vi "Tosca-Setup Imaging.vi"(0 "Imaging In":T1, 1 "Parent VI":refnum<vi>) -> (4 "Imaging Out":T1, 8 "Canceled?":bool)   [LabVIEW 2020]
uses:
  Typedefs/Tosca-Imaging.ctl
  Imaging VIs/Tosca-Imaging Mode.ctl
  Imaging VIs/Tosca-2P Config.ctl
  Sub VIs/Tosca-Globals.vi
panel:
  in  "Mode":enum16{"Off", "Widefield", "Two-photon"}(ring)
  in  "Tab Control":enum32{"Off", "Widefield", "Two-photon"}(tab)
  in  "Frame trigger":enum16{"Digital output", "Analog output"}(ring)
  in  "Destination":u16(ring) items=["Signal 1", "Frame Out", "Signal 2"]
  in  "Frame rate":dbl format="%#_g Hz"
  in  "TrigSrc":u16(ring) caption="Trigger source" items=["Default", "/PXI1Slot2/PFI0", "/PXI1Slot3/PFI0", "/PXI1Slot3/PFI1", "/PXI1Slot3/PFI2", "/PXI1Slot3/PFI3", "/PXI1Slot3/PFI4", "/PXI1Slot3/PFI5", "/PXI1Slot3/PFI6", "/PXI1Slot3/PFI7", "/PXI1Slot3/PFI8", "/PXI1Slot3/PFI9", "/PXI1Slot3/PFI10", "/PXI1Slot3/PFI11", "/PXI1Slot3/PFI12", "/PXI1Slot3/PFI13", "/PXI1Slot3/PFI14", "/PXI1Slot3/PFI15", "/PXI1Slot4/PFI0", "/PXI1Slot4/PFI1", "/PXI1Slot4/PFI2", "/PXI1Slot4/PFI3", "/PXI1Slot4/PFI4", "/PXI1Slot4/PFI5", "/PXI1Slot4/PFI6", "/PXI1Slot4/PFI7", "/PXI1Slot4/PFI8", "/PXI1Slot4/PFI9", "/PXI1Slot4/PFI10", "/PXI1Slot4/PFI11", "/PXI1Slot4/PFI12", "/PXI1Slot4/PFI13", "/PXI1Slot4/PFI14", "/PXI1Slot4/PFI15"]
  in  "Terminal":u16(ring) items=["Default", "PFI0", "PFI1", "PFI2", "PFI3", "PFI4", "PFI5", "PFI6", "PFI7", "PFI8", "PFI9", "PFI10", "PFI11", "PFI12", "PFI13", "PFI14", "PFI15"]
  in  "Device":u16(ring) caption="Frame tracker" items=["PXI1Slot3", "PXI1Slot4"]
  out "exit signal":bool
  in  "Cancel":bool
  in  "OK":bool
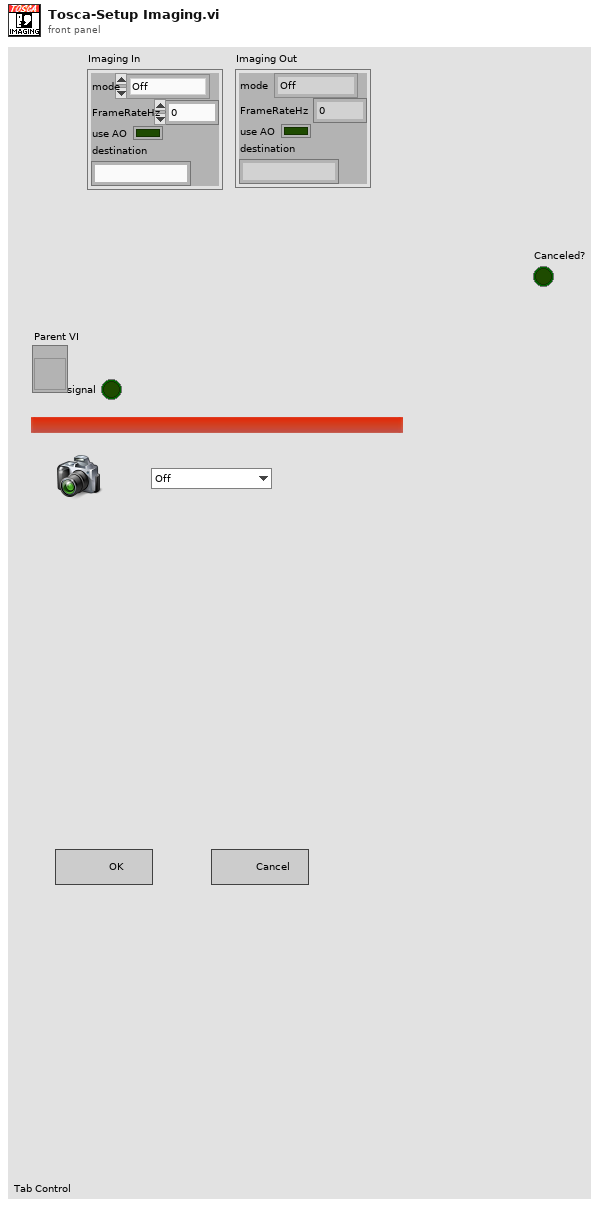
[diagram p1: front panel]
types:
  T1 = typedef "Tosca-Imaging.ctl" = cluster{"mode":T2, "FrameRateHz":dbl, "use AO":bool, "destination":string}
  T2 = typedef "Tosca-Imaging Mode.ctl" = enum16{"Off", "Widefield", "Two-photon"}
  T3 = typedef "Tosca-2P Config.ctl" = cluster{"Frame tracker":string, "Terminal":string, "Trigger source":string}
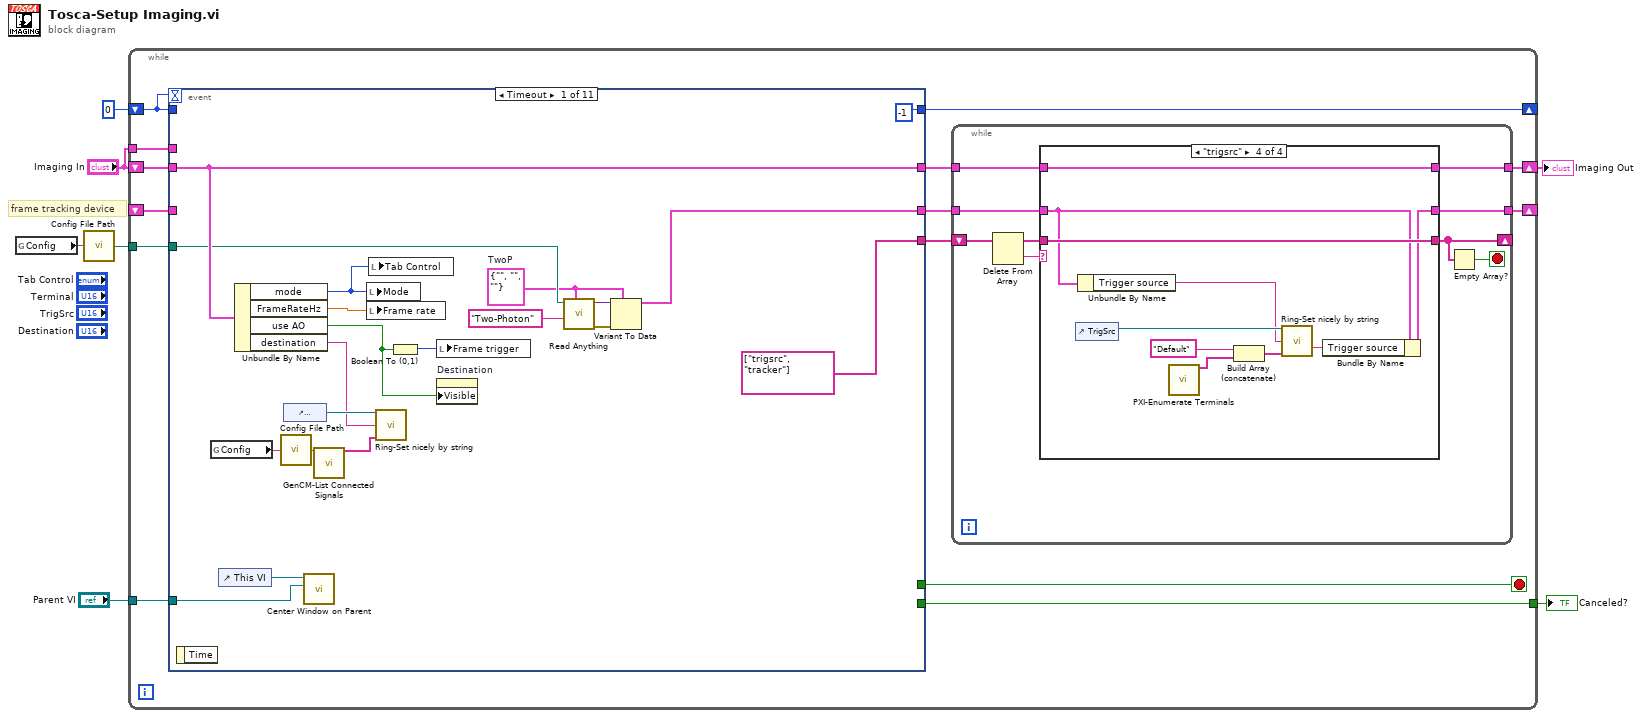
[diagram p0: block diagram]
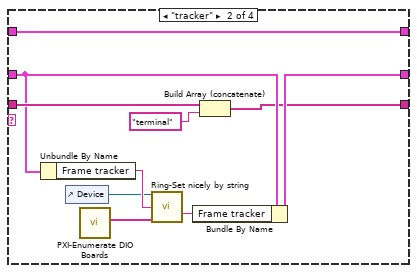
[diagram p3: hidden frame]
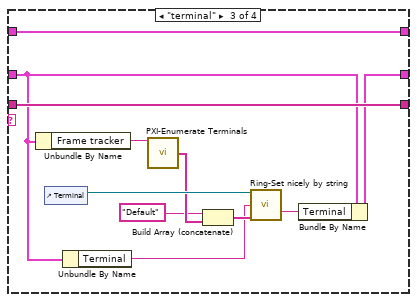
[diagram p4: hidden frame]
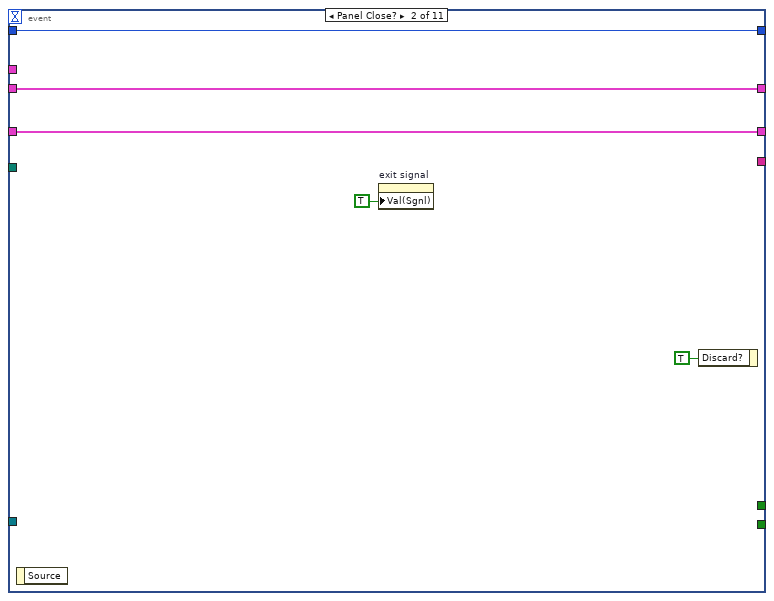
[diagram p5: hidden frame]
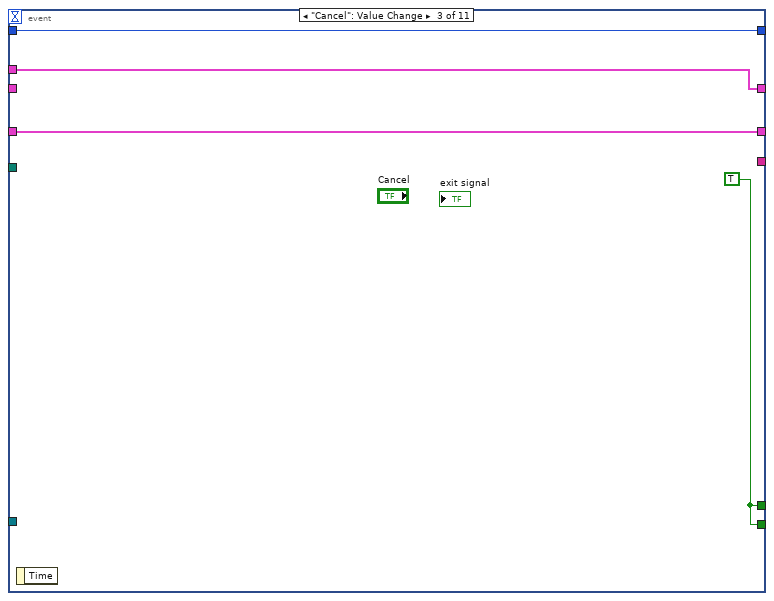
[diagram p6: hidden frame]
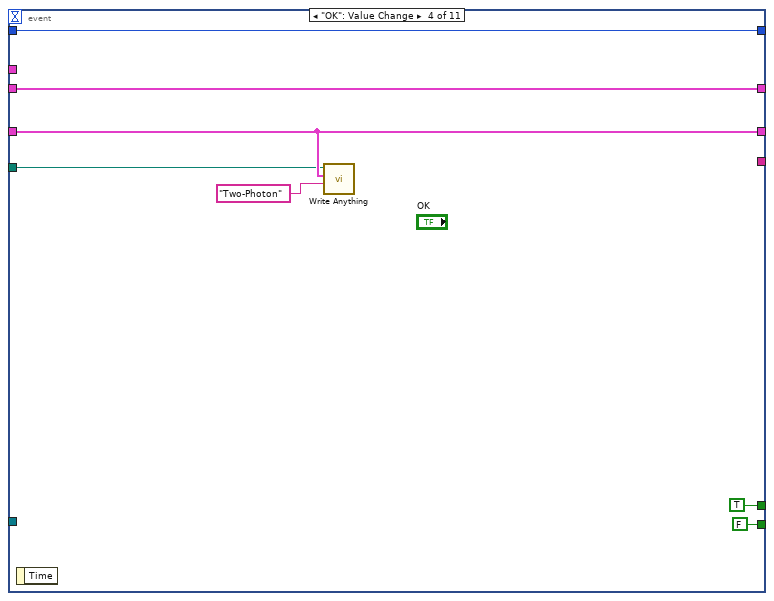
[diagram p7: hidden frame]
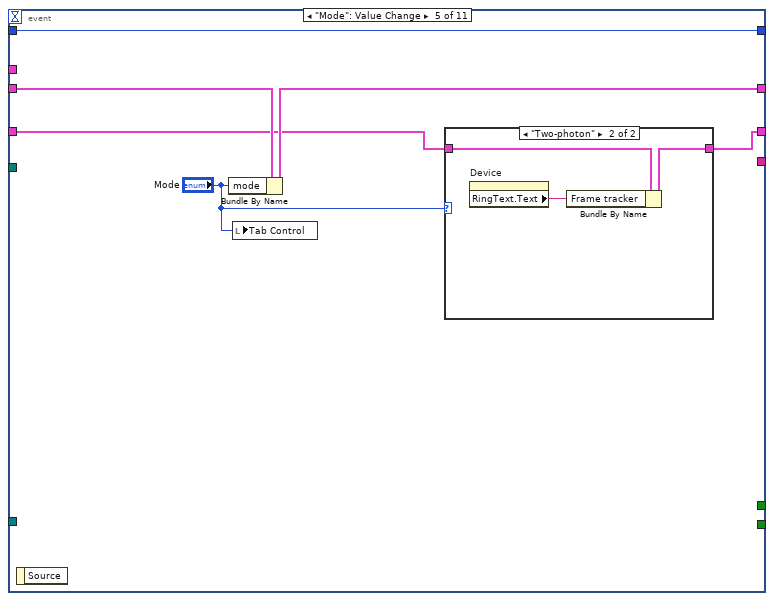
[diagram p8: hidden frame]
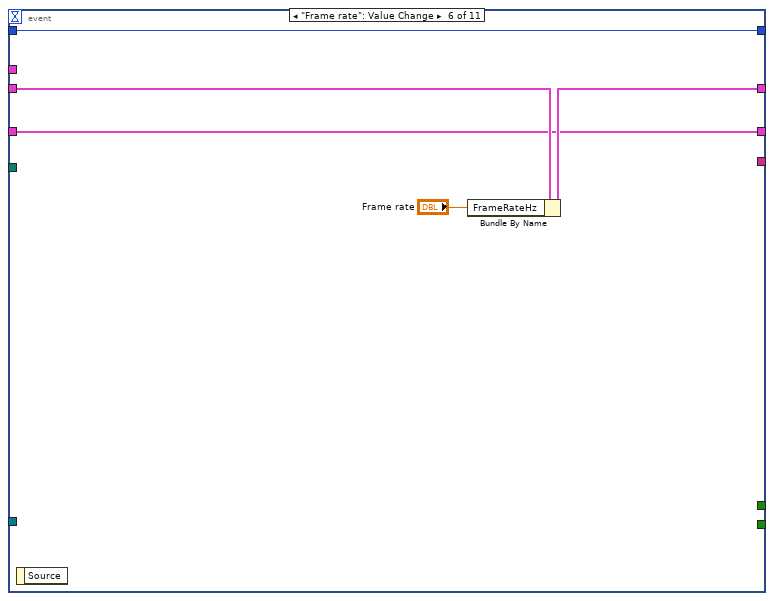
[diagram p10: hidden frame]
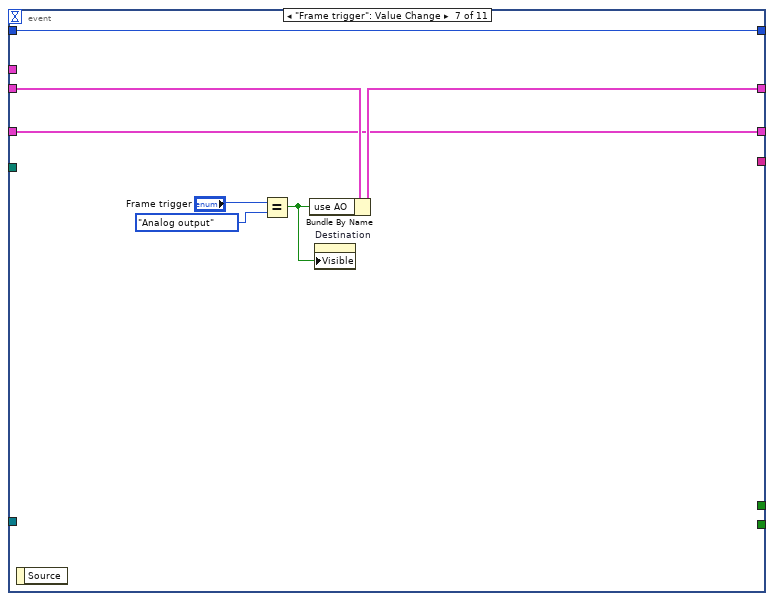
[diagram p11: hidden frame]
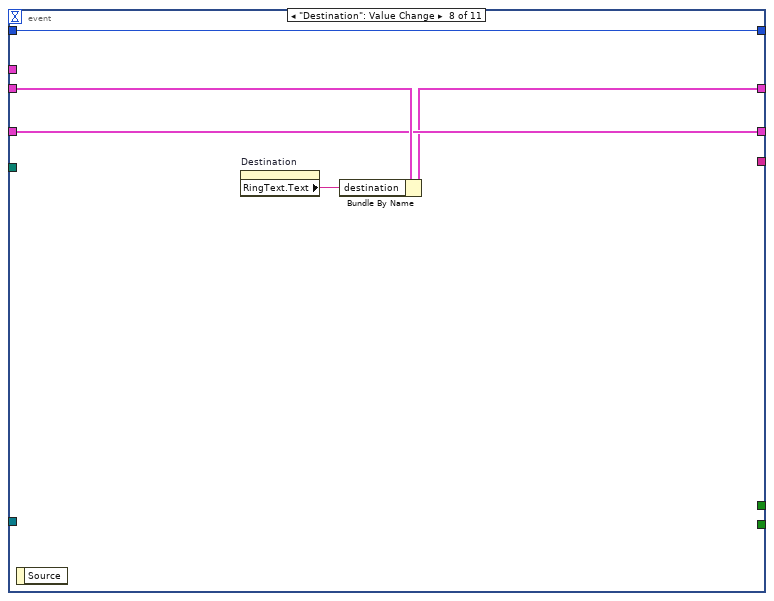
[diagram p12: hidden frame]
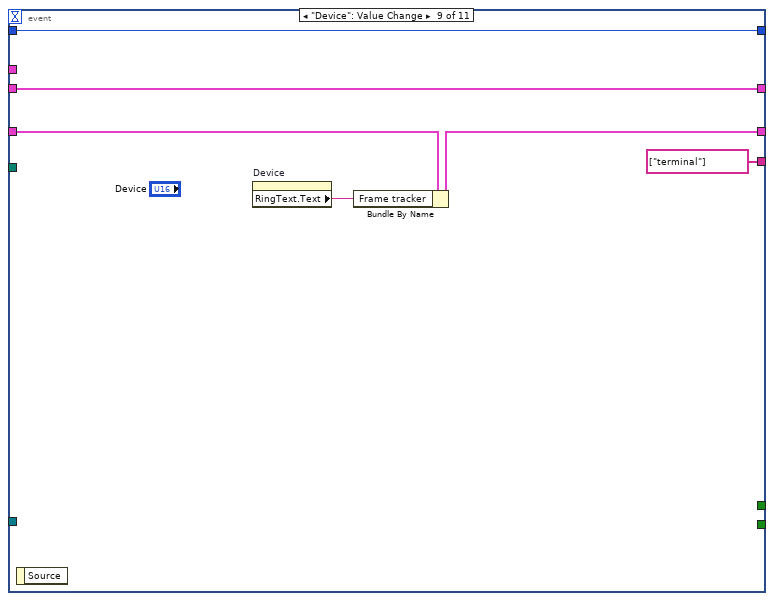
[diagram p13: hidden frame]
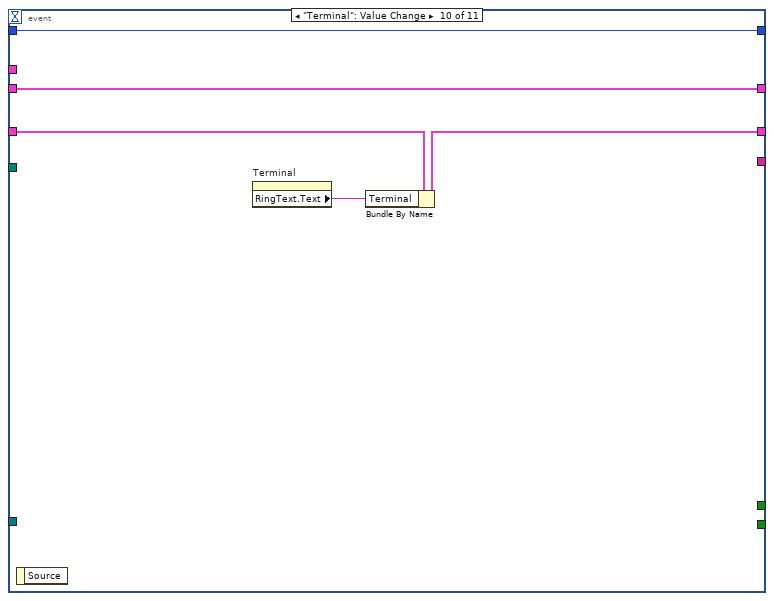
[diagram p14: hidden frame]
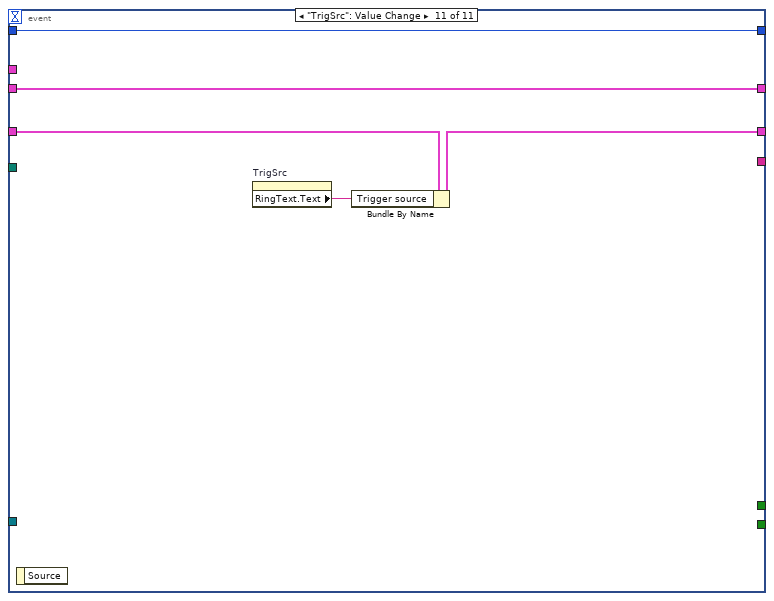
[diagram p15: hidden frame]
diagram:
  # "frame tracking device"
  n1 = global read "Tosca-Globals.vi" "Config"() -> (w1:string)
  n2 = call "Config File Path.vi"("AppName"=w1) -> ("Default config file name"=w4:path)
  n3 = while {
    shift-right: [w21] -> _
    shift-left: 0 -> [w17]
    tunnel: [w19] -> w5
    shift-right: [w12] -> w6
    shift-left: "Imaging In" -> [w18]
    tunnel: w4 -> [w8]
    shift-right: [w11] -> _
    shift-left: _ -> [w16]
    tunnel: "Imaging In" -> [w15]
    tunnel: "Parent VI" -> [w9]
    stop <- w20 stop-if-true
    n4 = event shown="[0] Timeout" {
      selector: _ -> [_ _ _ _ _ _ _ _ _ _ _]
      dyn-events: _ -> [_ _ _ _ _ _ _ _ _ _ _]
      timeout: w17 -> [_ _ _ _ _ _ _ _ _ _ _]
      tunnel: [-1 w89 w91 w97 w106 w115 w122 w127 w133 w138 w143] -> w21
      tunnel: w18 -> [w83 w88 _ w100 w105 w114 w121 w126 w132 w137 w142]
      tunnel: [w83 w88 w92 w100 w104 w113 w120 w124 w132 w137 w142] -> w14
      tunnel: [_ _ w93 TRUE _ _ _ _ _ _ _] -> w20
      tunnel: [_ _ w93 FALSE _ _ _ _ _ _ _] -> w19
      tunnel: w15 -> [_ _ w92 _ _ _ _ _ _ _ _]
      tunnel: w17 -> [_ w89 w91 w97 w106 w115 w122 w127 w133 w138 w143]
      tunnel: w8 -> [w79 _ _ w94 _ _ _ _ _ _ _]
      tunnel: [w75 w85 w90 w95 w101 w111 w119 w125 w130 w135 w140] -> w13
      tunnel: w16 -> [_ w85 w90 w95 w103 w111 w119 w125 w131 w136 w141]
      tunnel: [string[] ["trigsrc", "tracker"] _ _ _ _ _ _ _ string[] ["terminal"] _ _] -> w10
      tunnel: w9 -> [w72 _ _ _ _ _ _ _ _ _ _]
      event Timeout {
        w76 = T3 {"Frame tracker"="", "Terminal"="", "Trigger source"=""}  # TwoP
        n5 = event-data() -> ()  [unwired: 1 in, 1 out]
        n6 = global read "Tosca-Globals.vi" "Config"() -> (w68:string)
        n7 = control-ref of="This VI"() -> (w73:refnum<vi>)
        n8 = Unbundle By Name(w83) -> ("mode"=w81:T2, "FrameRateHz"=w82:dbl, "use AO"=w65:bool, "destination"=w69:string)
        n9 = call "Config File Path.vi"("AppName"=w68) -> ("Default config file name"=w67:path)
        n10 = control-ref of="Destination"() -> (w70:refnum<vi>)
        n11 = call "Center Window on Parent.vi"("Parent VI"=w72, "VI in"=w73) -> ()  [unwired: 8 in, 2 out]
        n12 = call "GenCM-List Connected Signals.vi"("Path"=w67) -> ("Analog Outputs"=w66:string[])  [unwired: 10 in, 4 out]
        n13 = local write "Mode"(w81) -> ()
        n14 = local write "Frame rate"(w82) -> ()
        n15 = local write "Tab Control"(w81) -> ()
        n16 = call "Ring-Set nicely by string.vi"("Ring in"=w70, "Device"=w69, "Strings []"=w66) -> ()  [unwired: 8 in, 5 out]
        n17 = Boolean To (0,1)(Boolean=w65) -> (0, 1=w71:i16)
        n18 = local write "Frame trigger"(w71) -> ()
        n19 = property on="Destination" class="Ring (strict)"("Visible"=w65) -> ()  [unwired: 2 in, 2 out]
        n20 = call "Read Anything.vi"("Type of Anything"=w76, "Section Name (Name of \"Type of Anything\")"="Two-Photon" ("Section Name (Name of \"Type of Anything\")"), "Path (dialog)"=w79) -> ("Error Out"=w80:errorcluster, "Anything"=w78:variant)  [unwired: 6 in, 1 out]
        n21 = Variant To Data(error in=w80, type=w76, Variant=w78) -> (data=w75:T3)  [unwired: 1 out]
      }
      event Panel Close? {
        n22 = event-data() -> ()  [unwired: 1 in, 1 out]
        n23 = property on="exit signal" class="Bool (strict)"("Val(Sgnl)"=TRUE ("Value (Signaling)")) -> ()  [unwired: 2 in, 2 out]
        n24 = event-data("Discard?"=TRUE) -> ()  [unwired: 1 in, 1 out]
      }
      event "Cancel": Value Change {
        w93 = TRUE
        n25 = event-data() -> ()  [unwired: 1 in, 1 out]
      }
      event "OK": Value Change {
        n26 = event-data() -> ()  [unwired: 1 in, 1 out]
        n27 = call "Write Anything.vi"("Section Name (Name of \"Anything\")"="Two-Photon" ("Section Name (Name of \"Type of Anything\")"), "Anything"=w95, "Path (dialog)"=w94) -> ()  [unwired: 7 in, 2 out]
      }
      event "Mode": Value Change {
        n28 = event-data() -> ()  [unwired: 1 in, 1 out]
        n29 = Bundle By Name(cluster=w105, "mode"="Mode") -> (w104:T1)
        n30 = local write "Tab Control"("Mode") -> ()
        n31 = case shown="\"Two-photon\"" "Mode" {
          tunnel: w103 -> [w107 w110]
          tunnel: [w107 w109] -> w101
          frame "Off", Default {
          }
          frame "Two-photon" {
            n32 = property on="Device" class="Ring (strict)"() -> ("RingText.Text"=w108:string)  [unwired: 2 in, 2 out]
            n33 = Bundle By Name(cluster=w110, "Frame tracker"=w108) -> (w109:T3)
          }
        }
      }
      event "Frame rate": Value Change {
        n34 = event-data() -> ()  [unwired: 1 in, 1 out]
        n35 = Bundle By Name(cluster=w114, "FrameRateHz"="Frame rate") -> (w113:T1)
      }
      event "Frame trigger": Value Change {
        n36 = event-data() -> ()  [unwired: 1 in, 1 out]
        n37 = Equal?(x="Frame trigger", y=enum16{"Digital output", "Analog output"}."Analog output") -> (x = y?=w116:bool)
        n38 = Bundle By Name(cluster=w121, "use AO"=w116) -> (w120:T1)
        n39 = property on="Destination" class="Ring (strict)"("Visible"=w116) -> ()  [unwired: 2 in, 2 out]
      }
      event "Destination": Value Change {
        n40 = event-data() -> ()  [unwired: 1 in, 1 out]
        n41 = property on="Destination" class="Ring (strict)"() -> ("RingText.Text"=w123:string)  [unwired: 2 in, 2 out]
        n42 = Bundle By Name(cluster=w126, "destination"=w123) -> (w124:T1)
      }
      event "Device": Value Change {
        n43 = event-data() -> ()  [unwired: 1 in, 1 out]
        n44 = property on="Device" class="Ring (strict)"() -> ("RingText.Text"=w129:string)  [unwired: 2 in, 2 out]
        n45 = Bundle By Name(cluster=w131, "Frame tracker"=w129) -> (w130:T3)
      }
      event "Terminal": Value Change {
        n46 = event-data() -> ()  [unwired: 1 in, 1 out]
        n47 = property on="Terminal" class="Ring (strict)"() -> ("RingText.Text"=w134:string)  [unwired: 2 in, 2 out]
        n48 = Bundle By Name(cluster=w136, "Terminal"=w134) -> (w135:T3)
      }
      event "TrigSrc": Value Change {
        n49 = event-data() -> ()  [unwired: 1 in, 1 out]
        n50 = property on="TrigSrc" class="Ring (strict)"() -> ("RingText.Text"=w139:string)  [unwired: 2 in, 2 out]
        n51 = Bundle By Name(cluster=w141, "Trigger source"=w139) -> (w140:T3)
      }
    }
    n52 = while {
      tunnel: w14 -> [w30]
      tunnel: w13 -> [w29]
      tunnel: [w28] -> w12
      tunnel: [w27] -> w11
      shift-right: [w23] -> _
      shift-left: w10 -> [w26]
      stop <- w22 stop-if-true
      n53 = Delete From Array(array=w26) -> (deleted portion=w24:string, array with subset deleted=w25:string[])  [unwired: 2 in]
      n54 = case shown="\"trigsrc\"" w24 {
        tunnel: w30 -> [w32 w43 w54 w64]
        tunnel: w29 -> [w33 w38 w47 w59]
        tunnel: [w32 w43 w54 w64] -> w28
        tunnel: [w33 w37 w45 w57] -> w27
        tunnel: w25 -> [w31 w42 w53 w63]
        tunnel: [w31 w35 w53 w63] -> w23
        frame "", Default {
        }
        frame "tracker" {
          n55 = Unbundle By Name(w38) -> ("Frame tracker"=w41:string)
          n56 = control-ref of="Device"() -> (w40:refnum<vi>)
          n57 = call "PXI-Enumerate DIO Boards.vi"() -> ("Devices"=w39:tag[])  [unwired: 10 in, 1 out]
          n58 = call "Ring-Set nicely by string.vi"("Ring in"=w40, "Device"=w41, "Strings []"=w39) -> ("Selection"=w36:string)  [unwired: 8 in, 4 out]
          n59 = Bundle By Name(cluster=w38, "Frame tracker"=w36) -> (w37:T3)
          n60 = Build Array (concatenate)(w42, "terminal") -> (w35:string[])
        }
        frame "terminal" {
          n61 = Unbundle By Name(w47) -> ("Frame tracker"=w52:string)
          n62 = control-ref of="Terminal"() -> (w51:refnum<vi>)
          n63 = Unbundle By Name(w47) -> ("Terminal"=w46:string)
          n64 = call "PXI-Enumerate Terminals.vi"("ActiveDev"=w52) -> ("Terminals"=w50:string[])  [unwired: 12 in, 2 out]
          n65 = Build Array (concatenate)("Default", w50) -> (w48:string[])
          n66 = call "Ring-Set nicely by string.vi"("Ring in"=w51, "Device"=w46, "Strings []"=w48) -> ("Selection"=w44:string)  [unwired: 8 in, 4 out]
          n67 = Bundle By Name(cluster=w47, "Terminal"=w44) -> (w45:T3)
        }
        frame "trigsrc" {
          n68 = control-ref of="TrigSrc"() -> (w62:refnum<vi>)
          n69 = Unbundle By Name(w59) -> ("Trigger source"=w58:string)
          n70 = call "PXI-Enumerate Terminals.vi"() -> ("Full"=w55:string[])  [unwired: 13 in, 2 out]
          n71 = Build Array (concatenate)("Default", w55) -> (w60:string[])
          n72 = call "Ring-Set nicely by string.vi"("Ring in"=w62, "Device"=w58, "Strings []"=w60) -> ("Selection"=w56:string)  [unwired: 8 in, 4 out]
          n73 = Bundle By Name(cluster=w59, "Trigger source"=w56) -> (w57:T3)
        }
      }
      n74 = Empty Array?(array=w23) -> (empty?=w22:bool)
    }
  }
  "Imaging Out" <- w6
  "Canceled?" <- w5
